vi "getLogString.vi"(8 "error in (no error)":errorcluster, 11 "Log.lvclass in":refnum<class "Log.lvclass">) -> (0 "error out":errorcluster, 2 "logString":string, 3 "Log.lvclass out":refnum<class "Log.lvclass">)   [LabVIEW 2011, in "Tools.lvlib" / "xml.lvlib" / "Log.lvclass"]
uses:
  Log.lvclass
  Log.lvclass/Log.ctl
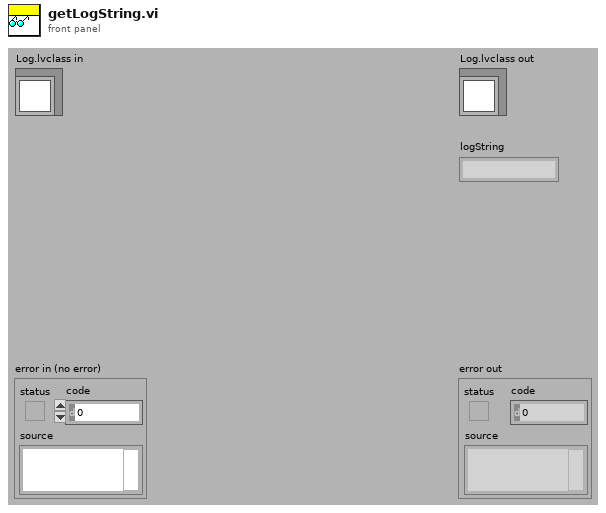
[diagram p1: front panel]
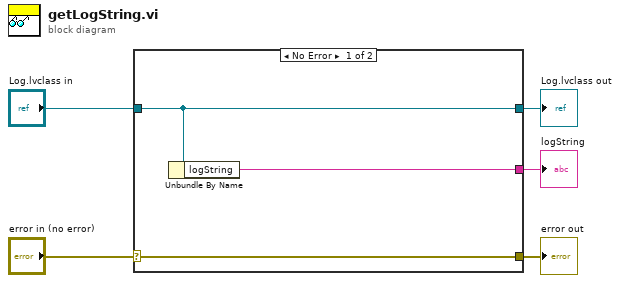
[diagram p0: block diagram]
diagram:
  n1 = case shown="No Error" "error in (no error)" {
    selector: "error in (no error)" -> [w8 w9]
    tunnel: [w8 w9] -> w4
    tunnel: [w7 w10] -> w2
    tunnel: "Log.lvclass in" -> [w7 w10]
    tunnel: [w6 _] -> w1
    frame No Error {
      n2 = Unbundle By Name(w7) -> ("logString"=w6:string)
    }
    frame Error {
    }
  }
  "error out" <- w4
  "Log.lvclass out" <- w2
  "logString" <- w1
